vi "GUIAS CURVAS EM FUNÇÃO DO RAIO.vi"() -> ()   [LabVIEW 2014]
uses:
  <vilib>/Platform/TimedLoop/XDataNode/timing_clust.ctl
  <vilib>/Platform/TimedLoop/XDataNode/nitl_modes.ctl
  <vilib>/Platform/TimedLoop/XDataNode/wakeup.ctl
  <vilib>/Instr/_visa.llb/VISA Configure Serial Port (Instr).vi
  <vilib>/Platform/TimedLoop/XDataNode/XDataNode.xnode
  <userlib>/Newport ESP301/Newport ESP301.lvlib
  <vilib>/Platform/TimedLoop/XDataNode/XDNodeRunTimeDep.lvlib
panel:
  in  "dGuia":dbl=100.0 format="%#_6f"
  out "theta":ext
  out "d (um)":dbl
  in  "Velocity":dbl=1.0
  out "In.Curva":dbl
  out "Yin":dbl format="%.6g"
  out "Xin":dbl format="%.6g"
  in  "d":dbl=100.0
  in  "Raios":dbl[](array[numeric])=[50.0]
  in  "In.Curva":dbl=1.0
  in  "Refresh Button":bool
  out "XY Graph":cluster{dbl[], dbl[]}(graph)={[0.0, 0.0, 0.0, 0.0, 0.0, 0.0, 0.0, 0.0, 0.0, 0.0, 0.0, 0.0, 0.0, 0.0, 0.0, 0.0, 0.0, 0.0, 0.0, 0.0, 0.0, 0.0, 0.0, 0.0, 0.0, 0.0, 0.0, 0.0, 0.0, 0.0, 0.0, 0.0, 0.0, 0.0, 0.0, 0.0, 0.0, 0.0, 0.0, 0.0, 0.0, 0.0, 0.0, 0.0, 0.0, 0.0, 0.0, 0.0, 0.0, 0.0, 0.0, 0.0, 0.0, 0.0, 0.0, 0.0, 0.0, 0.0, 0.0, 0.0, 0.0, 0.0, 0.0, 0.0, 0.0, 0.0, 0.0, 0.0, 0.0, 0.0, 0.0, 0.0, 0.0, 0.0, 0.0, 0.0], [4600.0, 4600.0, 4600.0, 4600.0, 4600.0, 4600.0, 4600.0, 4600.0, 4600.0, 4600.0, 4600.0, 4600.0, 4600.0, 4600.0, 4600.0, 4600.0, 4600.0, 4600.0, 4600.0, 4600.0, 4600.0, 4600.0, 4600.0, 4600.0, 4600.0, 4600.0, 4600.0, 4690.0, 4802.5, 4800.5, 4799.5, 4799.5, 4799.5, 4800.0, 4800.0, 4800.0, 4800.0, 4800.0, 4800.0, 4800.0, 4800.0, 4800.0, 4800.0, 4800.0, 4995.5, 5001.5, 5000.5, 5000.0, 5000.0, 4999.5, 4999.5, 5000.0, 5000.0, 5000.0, 5000.0, 5000.0, 5000.0, 5000.0, 5000.0, 5000.0, 5000.0, 5000.0, 5000.0, 5000.0, 5000.0, 5000.0, 5000.0, 5000.0, 5000.0, 5000.0, 5000.0, 5000.0, 5000.0, 5000.0, 5000.0, 5000.0]}
  out "Y (um)":dbl format="%.1f"
  out "X (mm)":dbl format="%.2g"
  out "PROGRESSÃO":i32
  in  "Defina Home":bool
  in  "Iniciar":bool
  in  "Stop Button":bool
  in  "L":dbl=5.0 format="%.1f"
  in  "N_Guias":i32=1
  # "TAMANHO DA AMOSTRA (mm)"
  # "Velocidade (mm/s)"
  # "DISTÂNCIA ENTRE ENTRADA E SAÍDA GUIA (um)"
  # "Número guias curvas"
  # "DISTÂNCIA ENTRE GUIAS (um)"
  # "Início da Curva (mm)"
  # "Raio (mm)"
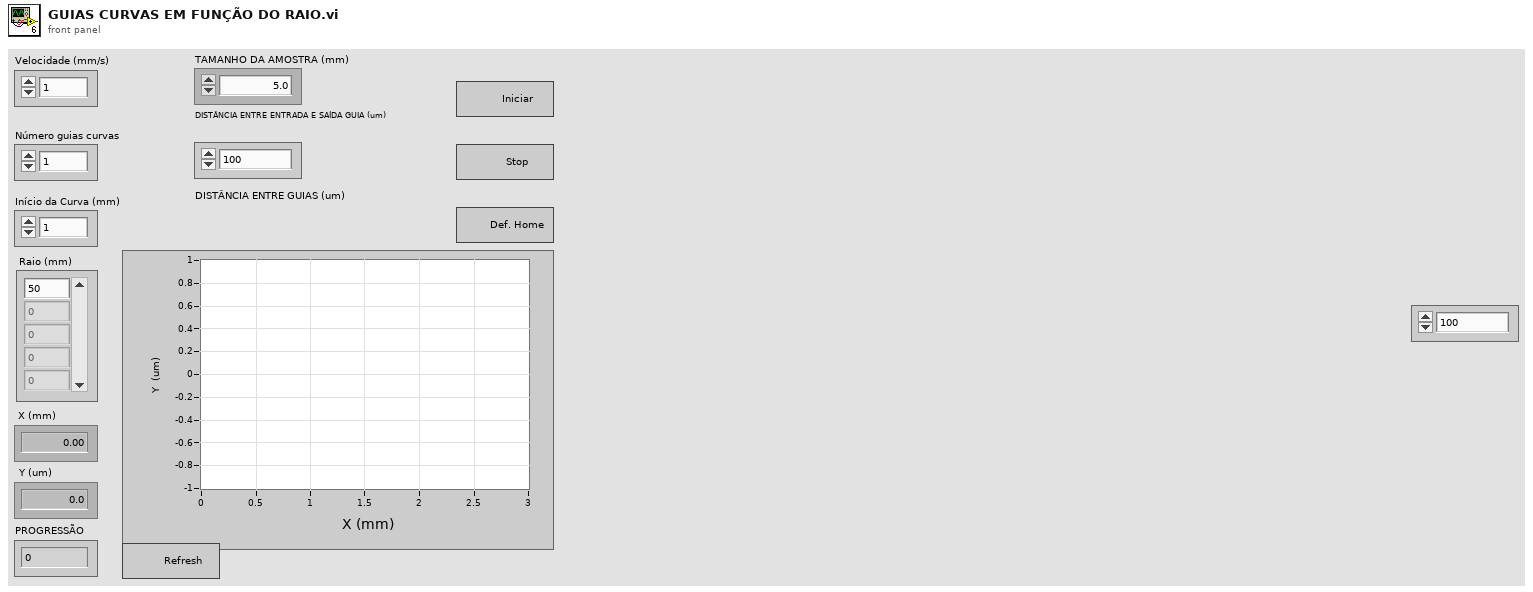
[diagram p1: front panel]
types:
  T1 = typedef "XDNodeRunTimeDep.lvlib/timing_clust.ctl" = cluster{"Expected End [f-1]":u64, "Actual End [f-1]":u64, "Finished Late? [f-1]":bool, "Expected End [i-1]":u64, "Actual End [i-1]":u64, "Finished Late? [i-1]":bool, "Expected Start [i]":u64, "Actual Start [i]":u64, "Expected Start [f]":u64, "Actual Start [f]":u64, "Source Name":string, "Structure Name":string, "Period":i64, "Deadline":i64, "Offset":i64, "Start":i64, "Priority":i32, "Timeout":i32, "Mode":T2, "Wakeup Reason":T3, "Error":errorcluster, "Source Type":string, "Secondary Source Type":string, "Global End Time":u64, "Global Start Time":u64, "Frame Duration":u64, "Iteration Duration":u64, "Assigned CPU":i32, "I/O Scan Engine Mode":u32}
  T2 = typedef "XDNodeRunTimeDep.lvlib/nitl_modes.ctl" = enum32{"No Change", "Process missed periods, maintain original phase", "Discard missed periods, maintain original phase", "Process missed periods, ignore original phase", "Discard missed periods, ignore original phase"}
  T3 = typedef "XDNodeRunTimeDep.lvlib/wakeup.ctl" = enum32{"Normal", "Aborted", "Asynchronous wakeup", "Timing source error", "Timed loop error", "Timeout"}
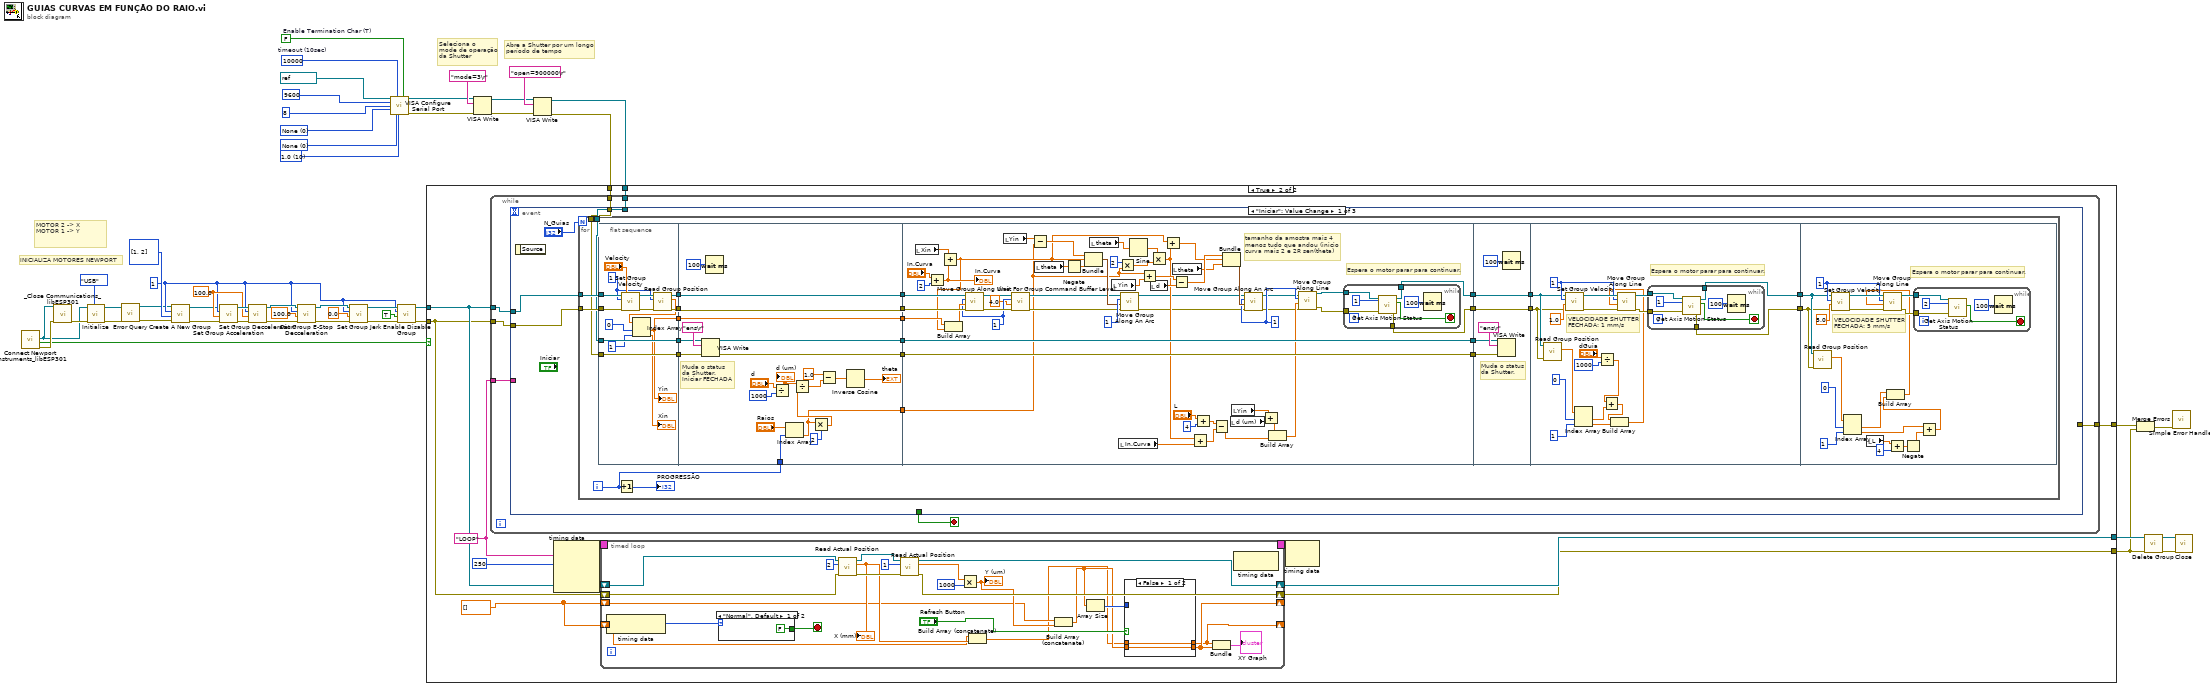
[diagram p0: block diagram]
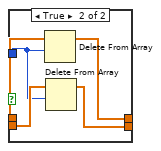
[diagram p3: hidden frame]
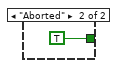
[diagram p4: hidden frame]
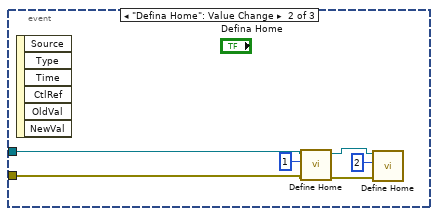
[diagram p5: hidden frame]
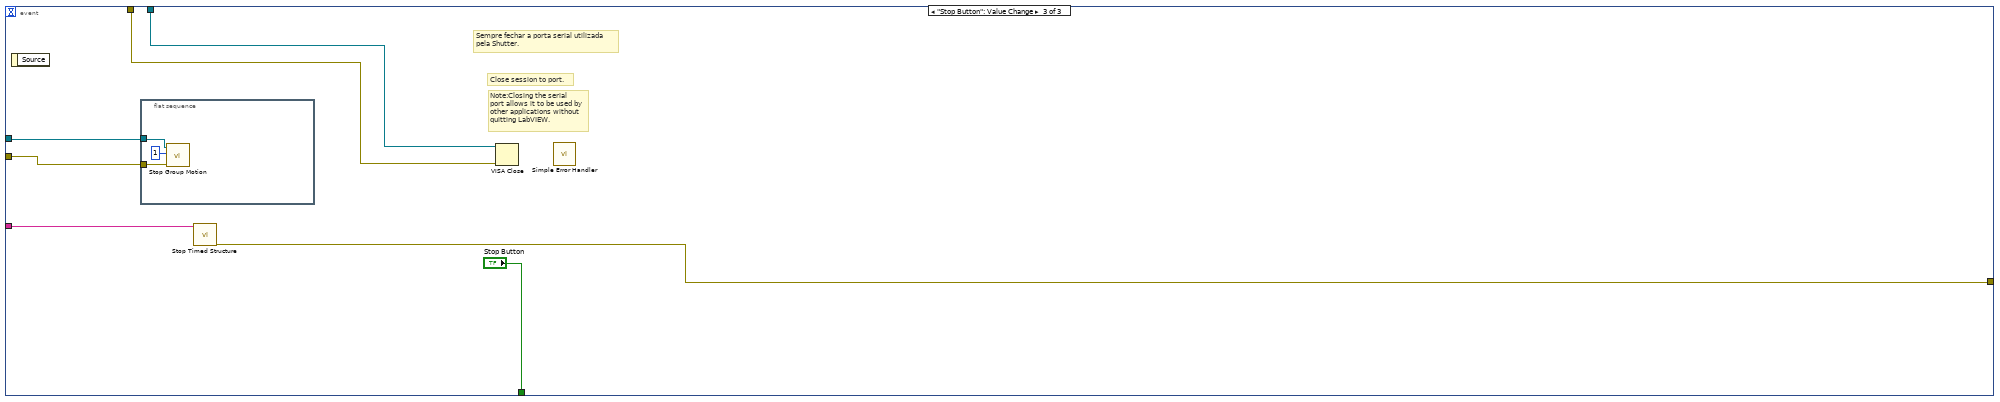
[diagram p6: hidden frame]
diagram:
  w13 = 1 ("Group #")
  w22 = 100.0 ("Acceleration (0 units/s²)")
  w39 = u16 0 items=["None", "Odd", "Even", "Mark", "Space"] ("parity")
  w42 = u16 10 items=["1.0"=10, "1.5"=15, "2.0"=20] ("stop bits")
  w43 = u16 0 items=["None"=0, "XON/XOFF"=1, "RTS/CTS"=2, "DTR/DSR"=4] ("flow control")
  w41 = FALSE  # Enable Termination Char (T)
  w40 = u32 10000  # timeout (10sec)
  # "MOTOR 2 -> X\nMOTOR 1 -> Y"
  # "Abre a Shutter por um longo\nperíodo de tempo"
  # "Seleciona o \nmode de operação\nda Shutter"
  # "INICIALIZA MOTORES NEWPORT"
  n1 = call <userlib>:"Connect Newport Instruments_libESP301.vi"() -> ("error (duplicate)"=w47:errorcluster, "Connected"=w45:bool, "VISA resource name (duplicate)"=w46:refnum<visa-resource-name>)  [unwired: 7 in, 2 out]
  n2 = call <userlib>:"_Close Communications_libESP301.vi"("Instrument Channel"=w46, "error in (no error)"=w47) -> ("error out"=w49:errorcluster)  [unwired: 13 in]
  n3 = call <userlib>:"Initialize.vi"("VISA resource name"=w46, "error in (no error)"=w49, "Serial Link (RS232)"=enum16{"RS232", "USB"}."USB") -> ("VISA resource name out"=w3:refnum<visa-resource-name>, "error out"=w4:errorcluster)  [unwired: 6 in]
  n4 = call <userlib>:"Error Query.vi"("error in (no error)"=w4, "VISA resource name"=w3) -> ("error out"=w1:errorcluster, "VISA resource name out"=w2:refnum<visa-resource-name>)  [unwired: 2 in, 2 out]
  n5 = call <userlib>:"Create A New Group.vi"("error in (no error)"=w1, "Axis Number"=i32[] [1, 2], "Group Number (1)"=w13, "VISA resource name"=w2) -> ("error out"=w5:errorcluster, "VISA resource name out"=w6:refnum<visa-resource-name>)  [unwired: 2 in]
  n6 = call <userlib>:"Set Group Acceleration.vi"("error in (no error)"=w5, "Acceleration (0 units/s²)"=w22, "Group Number (1)"=w13, "VISA resource name"=w6) -> ("error out"=w23:errorcluster, "VISA resource name out"=w24:refnum<visa-resource-name>)  [unwired: 2 in]
  n7 = call <userlib>:"Set Group Decceleration.vi"("error in (no error)"=w23, "Decceleration (0 units/s²)"=w22, "Group Number (1)"=w13, "VISA resource name"=w24) -> ("error out"=w18:errorcluster, "VISA resource name out"=w21:refnum<visa-resource-name>)  [unwired: 2 in]
  n8 = call <userlib>:"Set Group E-Stop Decceleration.vi"("error in (no error)"=w18, "E-Stop Decceleration (0 units/s²)"=100.0, "Group Number (1)"=w13, "VISA resource name"=w21) -> ("error out"=w17:errorcluster, "VISA resource name out"=w20:refnum<visa-resource-name>)  [unwired: 2 in]
  n9 = call <userlib>:"Set Group Jerk.vi"("error in (no error)"=w17, "Vector Jerk (0 units/s^3)"=0.0, "Group Number (1)"=w13, "VISA resource name"=w20) -> ("error out"=w16:errorcluster, "VISA resource name out"=w19:refnum<visa-resource-name>)  [unwired: 2 in]
  n10 = call-poly "VISA Configure Serial Port"("VISA resource name"=refnum<visa-resource-name> "COM6", "timeout (10sec)"=w40, "Enable Termination\nChar (T)"=w41, "baud rate (9600)"=u32 9600 ("baud rate"), "data bits (8)"=u16 8 ("data bits"), "parity (0:none)"=w39, "stop bits (10: 1 bit)"=w42, "flow control (0:none)"=w43) -> ("VISA resource name out"=w35:refnum<visa-resource-name>, "error out"=w34:errorcluster)  [unwired: 6 in]
  n11 = call <userlib>:"Enable Disable Group.vi"("error in (no error)"=w16, "Action (OFF)"=TRUE, "Group Number (1)"=w13, "VISA resource name"=w19) -> ("error out"=w11:errorcluster, "VISA resource name out"=w12:refnum<visa-resource-name>)  [unwired: 2 in]
  n12 = VISA Write(VISA resource name=w35, write buffer="mode=3\r", error in (no error)=w34) -> (VISA resource name out=w32:refnum<visa-resource-name>, error out=w31:errorcluster)  [unwired: 1 out]
  n13 = VISA Write(VISA resource name=w32, write buffer="open=900000\r", error in (no error)=w31) -> (VISA resource name out=w28:refnum<visa-resource-name>, error out=w27:errorcluster)  [unwired: 1 out]
  n14 = case shown="True" w45 {
    tunnel: w11 -> [w50 w52]
    tunnel: w12 -> [w51 w53]
    tunnel: [w51 w60] -> w10
    tunnel: [w50 w59] -> w8
    tunnel: [_ w57] -> w30
    tunnel: w28 -> [_ w56]
    tunnel: w27 -> [_ w55]
    frame False {
    }
    frame True {
      w54 = dbl[] []
      w58 = "LOOP" ("Structure Name")
      n15 = while {
        tunnel: w53 -> [w110]
        tunnel: w52 -> [w109]
        tunnel: w58 -> [w107]
        tunnel: [w106] -> w57
        tunnel: w56 -> [w105]
        tunnel: w55 -> [w104]
        stop <- w108 stop-if-true
        n16 = event shown="[0] \"Iniciar\": Value Change" {
          selector: _ -> [_ _ _]
          dyn-events: _ -> [_ _ _]
          timeout: _ -> [_ _ _]
          tunnel: w110 -> [w113 w301 w308]
          tunnel: w109 -> [w114 w300 w307]
          tunnel: [_ _ "Stop Button"] -> w108
          tunnel: w107 -> [_ _ w305]
          tunnel: [_ _ w304] -> w106
          tunnel: w105 -> [w112 _ w303]
          tunnel: w104 -> [w111 _ w302]
          event "Iniciar": Value Change {
            n17 = event-data() -> ()  [unwired: 1 in, 1 out]
            n18 = for {
              N: "N_Guias" -> [_]
              tunnel: w114 -> [w140]
              tunnel: w113 -> [w139]
              tunnel: w112 -> [w130]
              tunnel: w111 -> [w129]
              i -> [w119]
              n19 = flat-sequence {
                tunnel: w129 -> [w154]
                tunnel: w130 -> [w155]
                tunnel: w139 -> [w153]
                tunnel: w140 -> [w152]
                tunnel: [w147] -> w125
                tunnel: [w155] -> w124
                tunnel: [w154] -> w123
                tunnel: [w143] -> w121
                tunnel: [w148] -> w120
                tunnel: [w176] -> w138
                tunnel: [w175] -> w137
                tunnel: [w172] -> w136
                tunnel: [w171] -> w135
                tunnel: w125 -> [w176]
                tunnel: w124 -> [w170]
                tunnel: w123 -> [w169]
                tunnel: [w168] -> w122
                tunnel: w121 -> [w168]
                tunnel: w120 -> [w175]
                tunnel: w119 -> [w157]
                tunnel: [w156] -> w118
                tunnel: [w231] -> w127
                tunnel: [w230] -> w126
                tunnel: w135 -> [w230]
                tunnel: w136 -> [w231]
                tunnel: w137 -> [w228]
                tunnel: w138 -> [w227]
                tunnel: w122 -> [w207]
                tunnel: w118 -> [w185]
                tunnel: [w184] -> w117
                tunnel: [w183] -> w116
                tunnel: w127 -> [w242]
                tunnel: w126 -> [w241]
                tunnel: [w240] -> w132
                tunnel: [w239] -> w131
                tunnel: w117 -> [w239]
                tunnel: w116 -> [w240]
                tunnel: [w259] -> w134
                tunnel: w132 -> [w252]
                tunnel: w131 -> [w253]
                tunnel: [w258] -> w128
                tunnel: w134 -> [w278]
                tunnel: w128 -> [w277]
                frame #0 {
                  w141 = 1 ("Group Number (1)")
                  n20 = call <userlib>:"Set Group Velocity.vi"("error in (no error)"=w152, "Velocity (units/s)"="Velocity", "Group Number (1)"=w141, "VISA resource name"=w153) -> ("error out"=w149:errorcluster, "VISA resource name out"=w150:refnum<visa-resource-name>)  [unwired: 2 in]
                  n21 = call <userlib>:"Read Group Position.vi"("error in (no error)"=w149, "Group Number (1)"=w141, "VISA resource name"=w150) -> ("error out"=w147:errorcluster, "Position (units)"=w144:dbl[], "VISA resource name out"=w148:refnum<visa-resource-name>)  [unwired: 2 in]
                  n22 = Index Array(array=w144, index #1=0 ("index"), index #2=1 ("index")) -> (element #1=w143:dbl, element #2=→"Xin":dbl)
                  "Yin" <- w143
                }
                frame #1 {
                  # "Muda o status\nda Shutter.\nIniciar FECHADA"
                  n23 = VISA Write(VISA resource name=w170, write buffer="ens\r", error in (no error)=w169) -> (VISA resource name out=w172:refnum<visa-resource-name>, error out=w171:errorcluster)  [unwired: 1 out]
                  n24 = Wait (ms)(milliseconds to wait=u32 100) -> ()  [unwired: 1 out]
                  n25 = Divide(x="d", y=1000) -> (x/y=w163:dbl)
                  "d (um)" <- w163
                  n26 = Index Array(array="Raios", index=w157) -> (element=w156:dbl)
                  n27 = Multiply(x=w156, y=2) -> (x*y=w160:dbl)
                  n28 = Divide(x=w163, y=w160) -> (x/y=w166:dbl)
                  n29 = Subtract(x=1.0, y=w166) -> (x-y=w167:dbl)
                  n30 = Inverse Cosine(1:w167) -> (0:→"theta":dbl)
                }
                frame #2 {
                  w186 = 1 ("Group Number (1)")
                  w197 = 1 ("Axis (1)")
                  # "Espera o motor parar para continuar."
                  # "tamanho da amostra mais 4\nmenos tudo que andou (inicio \ncurva mais 2 e 2R sen(theta)"
                  n31 = local read "Xin"() -> (w224:dbl)
                  n32 = Add(x="In.Curva", y=2) -> (x+y=w208:dbl)
                  "In.Curva" <- w208
                  n33 = Add(x=w224, y=w208) -> (x+y=w206:dbl)
                  n34 = Build Array(w207, w206) -> (w205:dbl[])
                  n35 = call <userlib>:"Move Group Along Line.vi"("error in (no error)"=w227, "Position (0 units)"=w205, "Group Number (1)"=w197, "VISA resource name"=w228) -> ("error out"=w198:errorcluster, "VISA resource name out"=w199:refnum<visa-resource-name>)  [unwired: 2 in]
                  n36 = local read "Yin"() -> (w223:dbl)
                  n37 = call <userlib>:"Wait For Group Command Buffer Level.vi"("error in (no error)"=w198, "level in group via point buffer"=4.0, "Group Number (1)"=w197, "VISA resource name"=w199) -> ("error out"=w194:errorcluster, "VISA resource name out"=w195:refnum<visa-resource-name>)  [unwired: 2 in]
                  n38 = Subtract(x=w223, y=w185) -> (x-y=w222:dbl)
                  n39 = local read "theta"() -> (w192:ext)
                  n40 = Negate(x=w192) -> (-x=w193:ext)
                  n41 = Bundle(w222, w206, w193) -> (w221:cluster{dbl, dbl, ext})  [unwired: 1 in]
                  n42 = local read "theta"() -> (w191:ext)
                  n43 = local read "Yin"() -> (w216:dbl)
                  n44 = Multiply(x=2, y=w185) -> (x*y=w189:dbl)
                  n45 = local read "In.Curva"() -> (w211:dbl)
                  n46 = call <userlib>:"Move Group Along An Arc.vi"("error in (no error)"=w194, "Arc  Parameters"=w221, "Group Number (1)"=1, "VISA resource name"=w195) -> ("error out"=w181:errorcluster, "VISA resource name out"=w182:refnum<visa-resource-name>)  [unwired: 2 in]
                  n47 = Sine(x=w191) -> (sin(x)=w190:ext)
                  n48 = Add(x=w185, y=w216) -> (x+y=w217:dbl)
                  n49 = Multiply(x=w190, y=w189) -> (x*y=w188:ext)
                  n50 = local read "d"() -> (w218:dbl)
                  n51 = Add(x=w206, y=w188) -> (x+y=w214:ext)
                  n52 = local read "theta"() -> (w187:ext)
                  n53 = Subtract(x=w217, y=w218) -> (x-y=w220:dbl)
                  n54 = Add(x=w188, y=w211) -> (x+y=w209:ext)
                  n55 = Add(x="L", y=4) -> (x+y=w210:dbl)
                  n56 = Subtract(x=w210, y=w209) -> (x-y=w204:ext)
                  n57 = Bundle(w220, w214, "theta"=w187) -> (w219:cluster{dbl, ext, "theta":ext})  [unwired: 1 in]
                  n58 = local read "d (um)"() -> (w200:dbl)
                  n59 = local read "Yin"() -> (w201:dbl)
                  n60 = call <userlib>:"Move Group Along An Arc.vi"("error in (no error)"=w181, "Arc  Parameters"=w219, "Group Number (1)"=w186, "VISA resource name"=w182) -> ("error out"=w179:errorcluster, "VISA resource name out"=w180:refnum<visa-resource-name>)  [unwired: 2 in]
                  n61 = Add(x=w201, y=w200) -> (x+y=w203:dbl)
                  n62 = Build Array(w203, w204) -> (w202:ext[])
                  n63 = call <userlib>:"Move Group Along Line.vi"("error in (no error)"=w179, "Position (0 units)"=w202, "Group Number (1)"=w186, "VISA resource name"=w180) -> ("error out"=w177:errorcluster, "VISA resource name out"=w178:refnum<visa-resource-name>)  [unwired: 2 in]
                  n64 = while {
                    tunnel: [w235] -> w184
                    tunnel: [w234] -> w183
                    tunnel: w178 -> [w233]
                    tunnel: w177 -> [w232]
                    stop <- w237 stop-if-true
                    n65 = call <userlib>:"Get Axis Motion Status.vi"("error in (no error)"=w232, "Axis (1)"=1, "VISA resource name"=w233) -> ("error out"=w234:errorcluster, "Motion Done"=w237:bool, "VISA resource name out"=w235:refnum<visa-resource-name>)  [unwired: 2 in]
                    n66 = Wait (ms)(milliseconds to wait=u32 100) -> ()  [unwired: 1 out]
                  }
                }
                frame #3 {
                  # "Muda o status\nda Shutter."
                  n67 = VISA Write(VISA resource name=w242, write buffer="ens\r", error in (no error)=w241) -> ()  [unwired: 3 out]
                  n68 = Wait (ms)(milliseconds to wait=u32 100) -> ()  [unwired: 1 out]
                }
                frame #4 {
                  w257 = 1 ("Axis (1)")
                  # "Espera o motor parar para continuar."
                  # "VELOCIDADE SHUTTER\nFECHADA: 1 mm/s"
                  n69 = call <userlib>:"Read Group Position.vi"("error in (no error)"=w252, "VISA resource name"=w253) -> ("Position (units)"=w254:dbl[])  [unwired: 3 in, 2 out]
                  n70 = call <userlib>:"Set Group Velocity.vi"("error in (no error)"=w252, "Velocity (units/s)"=1.0 ("Base Velocity (0 units/s)"), "Group Number (1)"=w257, "VISA resource name"=w253) -> ("error out"=w263:errorcluster, "VISA resource name out"=w262:refnum<visa-resource-name>)  [unwired: 2 in]
                  n71 = Index Array(array=w254, index #1=0 ("index"), index #2=1 ("index")) -> (element #1=w247:dbl, element #2=w248:dbl)
                  n72 = Divide(x="dGuia", y=1000) -> (x/y=w246:dbl)
                  n73 = Add(x=w246, y=w247) -> (x+y=w249:dbl)
                  n74 = Build Array(w249, w248) -> (w245:dbl[])
                  n75 = call <userlib>:"Move Group Along Line.vi"("error in (no error)"=w263, "Position (0 units)"=w245, "Group Number (1)"=w257, "VISA resource name"=w262) -> ("error out"=w260:errorcluster, "VISA resource name out"=w261:refnum<visa-resource-name>)  [unwired: 2 in]
                  n76 = while {
                    tunnel: [w268] -> w259
                    tunnel: [w267] -> w258
                    tunnel: w260 -> [w266]
                    tunnel: w261 -> [w265]
                    stop <- w270 stop-if-true
                    n77 = call <userlib>:"Get Axis Motion Status.vi"("error in (no error)"=w266, "Axis (1)"=1, "VISA resource name"=w265) -> ("error out"=w267:errorcluster, "Motion Done"=w270:bool, "VISA resource name out"=w268:refnum<visa-resource-name>)  [unwired: 2 in]
                    n78 = Wait (ms)(milliseconds to wait=u32 100) -> ()  [unwired: 1 out]
                  }
                }
                frame #5 {
                  w282 = 1 ("Axis (1)")
                  # "Espera o motor parar para continuar."
                  # "VELOCIDADE SHUTTER\nFECHADA: 5 mm/s"
                  n79 = call <userlib>:"Read Group Position.vi"("error in (no error)"=w277, "VISA resource name"=w278) -> ("Position (units)"=w279:dbl[])  [unwired: 3 in, 2 out]
                  n80 = call <userlib>:"Set Group Velocity.vi"("error in (no error)"=w277, "Velocity (units/s)"=5.0 ("Base Velocity (0 units/s)"), "Group Number (1)"=w282, "VISA resource name"=w278) -> ("error out"=w289:errorcluster, "VISA resource name out"=w288:refnum<visa-resource-name>)  [unwired: 2 in]
                  n81 = Index Array(array=w279, index #1=0 ("index"), index #2=1 ("index")) -> (element #1=w276:dbl, element #2=w275:dbl)
                  n82 = local read "L"() -> (w286:dbl)
                  n83 = Add(x=w286, y=4) -> (x+y=w285:dbl)
                  n84 = Negate(x=w285) -> (-x=w274:dbl)
                  n85 = Add(x=w275, y=w274) -> (x+y=w273:dbl)
                  n86 = Build Array(w276, w273) -> (w272:dbl[])
                  n87 = call <userlib>:"Move Group Along Line.vi"("error in (no error)"=w289, "Position (0 units)"=w272, "Group Number (1)"=w282, "VISA resource name"=w288) -> ("error out"=w283:errorcluster, "VISA resource name out"=w284:refnum<visa-resource-name>)  [unwired: 2 in]
                  n88 = while {
                    tunnel: w283 -> [w292]
                    tunnel: w284 -> [w291]
                    stop <- w294 stop-if-true
                    n89 = call <userlib>:"Get Axis Motion Status.vi"("error in (no error)"=w292, "Axis (1)"=2, "VISA resource name"=w291) -> ("Motion Done"=w294:bool)  [unwired: 2 in, 2 out]
                    n90 = Wait (ms)(milliseconds to wait=u32 100) -> ()  [unwired: 1 out]
                  }
                }
              }
              n91 = Increment(x=w119) -> (x+1=→"PROGRESSÃO":i32)
            }
          }
          event "Defina Home": Value Change {
            n92 = event-data() -> ()  [unwired: 1 in, 6 out]
            n93 = call <userlib>:"Define Home.vi"("error in (no error)"=w300, "Axis (1)"=1, "VISA resource name"=w301) -> ("error out"=w296:errorcluster, "VISA resource name out"=w297:refnum<visa-resource-name>)  [unwired: 3 in]
            n94 = call <userlib>:"Define Home.vi"("error in (no error)"=w296, "Axis (1)"=2, "VISA resource name"=w297) -> ()  [unwired: 3 in, 2 out]
          }
          event "Stop Button": Value Change {
            # "Sempre fechar a porta serial utilizada\npela Shutter."
            # "Note:Closing the serial port allows it to be used by other applications without\nquitting LabVIEW."
            # "Close session to port."
            n95 = event-data() -> ()  [unwired: 1 in, 1 out]
            n96 = flat-sequence {
              tunnel: w308 -> [w311]
              tunnel: w307 -> [w310]
              frame #0 {
                n97 = call <userlib>:"Stop Group Motion.vi"("error in (no error)"=w310, "Group Number (1)"=1 ("Axis (1)"), "VISA resource name"=w311) -> ()  [unwired: 3 in, 2 out]
              }
            }
            n98 = call <vilib>:"Stop Timed Structure.vi"("name"=w305) -> ("error out"=w304:errorcluster)  [unwired: 10 in]
            n99 = VISA Close(VISA resource name=w303, error in (no error)=w302) -> ()  [unwired: 1 out]
            n100 = call <vilib>:"Simple Error Handler.vi"() -> ()  [unwired: 5 in, 5 out]
          }
        }
      }
      n101 = node-c288(w58, i64 250 ("Period")) -> (w63:T1)  [unwired: 2 in]
      n102 = timed-loop {
        timing: w63 -> [_]
        timing-out: [_] -> w62
        shift-right: [w80] -> w60
        shift-left: w53 -> [w85]
        shift-right: [w79] -> w59
        shift-left: w52 -> [w84]
        shift-right: [w65] -> _
        shift-left: w54 -> [w69]
        shift-right: [w64] -> _
        shift-left: w54 -> [w67]
        stop <- w77 stop-if-true
        n103 = node-c288() -> (w78:T3)  [unwired: 1 in]
        n104 = case shown="\"Normal\", Default" w78 {
          tunnel: [FALSE TRUE] -> w77
          frame "Normal", Default {
          }
          frame "Aborted" {
          }
        }
        n105 = call <userlib>:"Read Actual Position.vi"("error in (no error)"=w84, "Axis (1)"=2, "VISA resource name"=w85) -> ("error out"=w83:errorcluster, "Position (units)"=w76:dbl, "VISA resource name out"=w82:refnum<visa-resource-name>)  [unwired: 2 in]
        "X (mm)" <- w76
        n106 = call <userlib>:"Read Actual Position.vi"("error in (no error)"=w83, "Axis (1)"=1, "VISA resource name"=w82) -> ("error out"=w79:errorcluster, "Position (units)"=w73:dbl, "VISA resource name out"=w80:refnum<visa-resource-name>)  [unwired: 2 in]
        n107 = Multiply(x=w73, y=u32 1000) -> (x*y=w72:dbl)
        "Y (um)" <- w72
        n108 = Build Array (concatenate)(w67, w76) -> (w66:dbl[])
        n109 = Build Array (concatenate)(w69, w72) -> (w68:dbl[])
        n110 = Array Size(array=w68) -> (size(s)=w70:i32)
        n111 = case shown="False" "Refresh Button" {
          tunnel: [w88 w90] -> w64
          tunnel: w66 -> [w88 w93]
          tunnel: [w87 w89] -> w65
          tunnel: w68 -> [w87 w92]
          tunnel: w70 -> [_ w91]
          frame False {
          }
          frame True {
            n112 = Delete From Array(array=w93, length=w91) -> (array with subset deleted=w90:dbl[])  [unwired: 1 in, 1 out]
            n113 = Delete From Array(array=w92, length=w91) -> (array with subset deleted=w89:dbl[])  [unwired: 1 in, 1 out]
          }
        }
        n114 = Bundle(w64, w65) -> (→"XY Graph":cluster{dbl[], dbl[]})  [unwired: 1 in]
        n115 = node-c288() -> ()  [unwired: 1 in, 1 out]
      }
      n116 = node-c288(w62) -> ()  [unwired: 1 out]
    }
  }
  n117 = Merge Errors(w30, w8) -> (w29:errorcluster)
  n118 = call <userlib>:"Delete Group.vi"("error in (no error)"=w8, "VISA resource name"=w10) -> ("error out"=w7:errorcluster, "VISA resource name out"=w9:refnum<visa-resource-name>)  [unwired: 4 in]
  n119 = call <vilib>:"Simple Error Handler.vi"("error in (no error)"=w29) -> ()  [unwired: 1 in, 8 out]
  n120 = call <userlib>:"Close.vi"("error in (no error)"=w7, "VISA resource name"=w9) -> ()  [unwired: 9 in, 1 out]
